vi "FaceLandmarkToPoints.vi"(8 "error in (no error)":errorcluster, 11 "FaceLandmark":refnum<k24>) -> (0 "error out":errorcluster, 2 "FaceLandmarkArray":cluster{"item":T1, T2[]}[][](array[cluster]) {"item" items=["Chin", "LeftEyebrow", "RightEyebrow", "NoseBridge", "NoseTip", "LeftEye", "RightEye", "TopLip", "BottomLip", "Nose"]; "?"."Y" format="%.2f"; "?"."X" format="%.2f"})   [LabVIEW 2020, in "FaceRecognitionDotNet.lvlib" / "FaceRecognition.lvclass"]
uses:
  FaceRecognition.lvclass
  ctl/FacePart.ctl
  ctl/Point.ctl
  dll/FaceRecognitionDotNet.dll
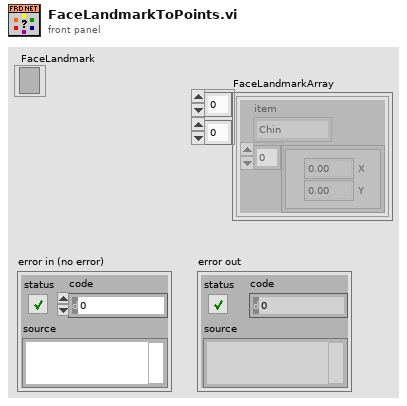
[diagram p1: front panel]
types:
  T1 = typedef "FaceRecognitionDotNet.lvlib/FaceRecognition.lvclass/FacePart.ctl" = i32
  T2 = typedef "FaceRecognitionDotNet.lvlib/FaceRecognition.lvclass/Point.ctl" = cluster{"X":sgl, "Y":sgl}
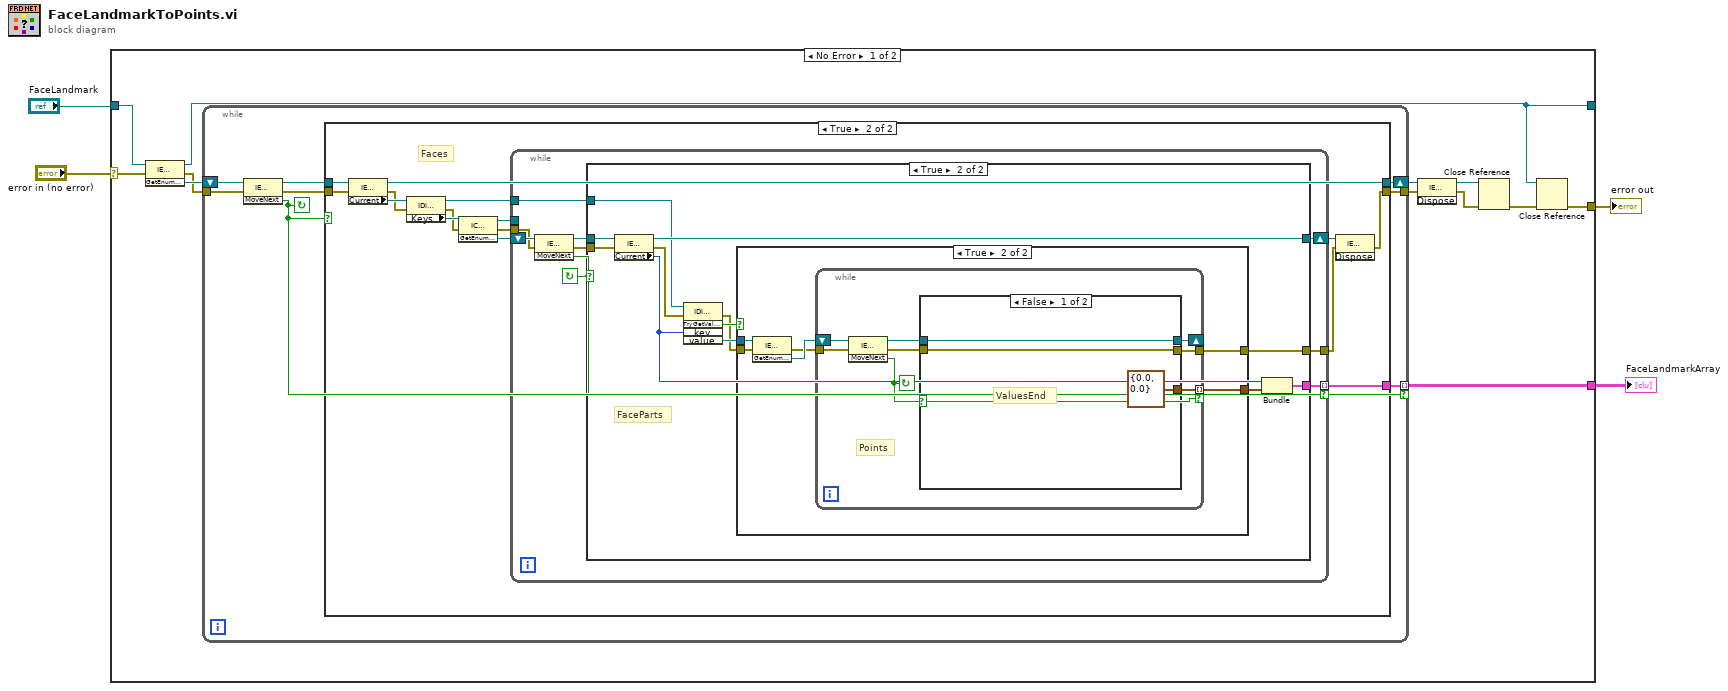
[diagram p0: block diagram]
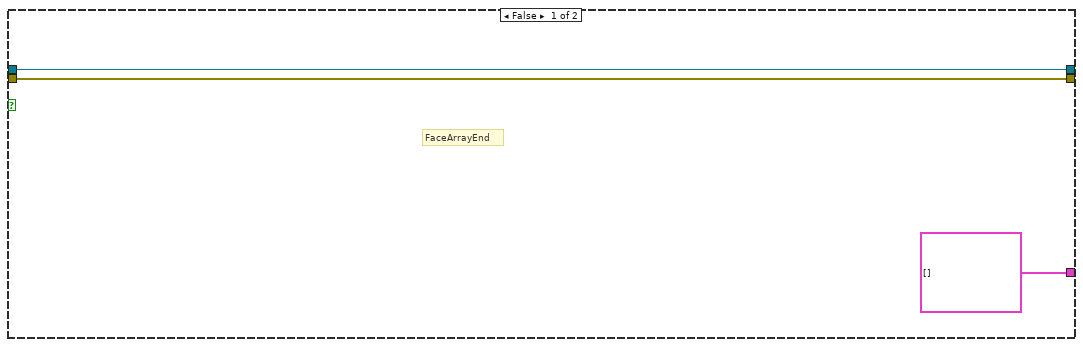
[diagram p2: hidden frame]
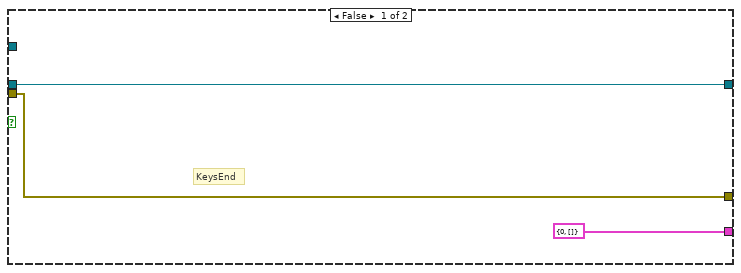
[diagram p3: hidden frame]
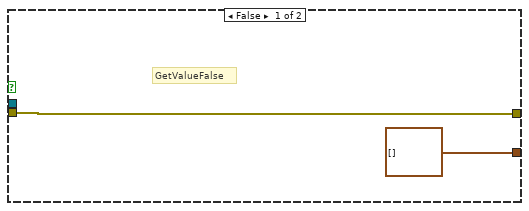
[diagram p4: hidden frame]
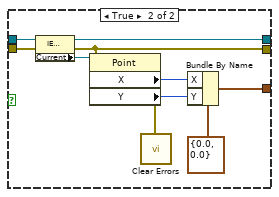
[diagram p5: hidden frame]
diagram:
  n1 = case shown="No Error" "error in (no error)" {
    selector: "error in (no error)" -> [w6 w97]
    tunnel: "FaceLandmark" -> [w16 w96]
    tunnel: [w13 _] -> w3
    tunnel: [w7 w97] -> w2
    tunnel: [w5 w96] -> _
    frame No Error {
      n2 = invoke class="IEnumerable`1[[System.Collectio" method="GetEnumerator"(reference=w16, error in=w6) -> (reference out=w5:refnum<k24>, error out=w14:errorcluster, "GetEnumerator"=w15:refnum<k24>)  [unwired: 1 in]
      n3 = while {
        tunnel: w14 -> [w21]
        shift-right: [w20] -> w12
        shift-left: w15 -> [w24]
        tunnel: [w19] -> w13 mode=indexing if=w18
        tunnel: [w17] -> w11
        stop <- w18 continue-if-true
        n4 = invoke class="IEnumerator`1[[System.Collectio" method="MoveNext"(reference=w24, error in=w21) -> (reference out=w23:refnum<k24>, error out=w22:errorcluster, "MoveNext"=w18:bool)  [unwired: 1 in]
        n5 = case shown="True" w18 {
          tunnel: w23 -> [w27 w42]
          tunnel: w22 -> [w25 w41]
          tunnel: [w27 w32] -> w20
          tunnel: [cluster{"item":i32, T2[]}[] [] w34] -> w19
          tunnel: [w25 w28] -> w17
          frame False {
            # "FaceArrayEnd"
          }
          frame True {
            # "Faces"
            n6 = property class="IEnumerator`1[[System.Collectio"(reference=w42, error in=w41) -> (reference out=w32:refnum<k24>, error out=w39:errorcluster, "Current"=w40:refnum<k24>)
            n7 = property class="IDictionary`2[[FaceRecognitionD"(reference=w40, error in=w39) -> (reference out=w33:refnum<k24>, error out=w35:errorcluster, "Keys"=w38:refnum<k24>)
            n8 = invoke class="ICollection`1[[FaceRecognitionD" method="GetEnumerator"(reference=w38, error in=w35) -> (reference out=w31:refnum<k24>, error out=w36:errorcluster, "GetEnumerator"=w37:refnum<k24>)  [unwired: 1 in]
            n9 = while {
              tunnel: w36 -> [w49]
              shift-right: [w47] -> w30
              shift-left: w37 -> [w51]
              tunnel: [w45] -> w34 mode=indexing if=w46
              tunnel: [w44] -> w29
              tunnel: w33 -> [w43]
              tunnel: w31 -> [_]
              stop <- w46 continue-if-true
              n10 = invoke class="IEnumerator`1[[FaceRecognitionD" method="MoveNext"(reference=w51, error in=w49) -> (reference out=w50:refnum<k24>, error out=w48:errorcluster, "MoveNext"=w46:bool)  [unwired: 1 in]
              n11 = case shown="True" w46 {
                tunnel: w50 -> [w54 w66]
                tunnel: w48 -> [w52 w65]
                tunnel: [w54 w64] -> w47
                tunnel: w43 -> [_ w63]
                tunnel: [cluster{"Current":i32, T2[]} {"Current"=0, []} w56] -> w45
                tunnel: [w52 w55] -> w44
                frame False {
                  # "KeysEnd"
                }
                frame True {
                  # "FaceParts"
                  n12 = property class="IEnumerator`1[[FaceRecognitionD"(reference=w66, error in=w65) -> (reference out=w64:refnum<k24>, error out=w62:errorcluster, "Current"=w57:i32)
                  n13 = invoke class="IDictionary`2[[FaceRecognitionD" method="TryGetValue"(reference=w63, error in=w62, "key"=w57) -> (error out=w59:errorcluster, "TryGetValue"=w60:bool, "value"=w61:refnum<k24>)  [unwired: 2 in, 2 out]
                  n14 = case shown="True" w60 {
                    tunnel: w61 -> [_ w74]
                    tunnel: [T2[] [] w69] -> w58
                    tunnel: w59 -> [w67 w71]
                    tunnel: [w67 w70] -> w55
                    frame False {
                      # "GetValueFalse"
                    }
                    frame True {
                      n15 = invoke class="IEnumerable`1[[FaceRecognitionD" method="GetEnumerator"(reference=w74, error in=w71) -> (error out=w72:errorcluster, "GetEnumerator"=w73:refnum<k24>)  [unwired: 1 in, 1 out]
                      n16 = while {
                        shift-right: [w80] -> _
                        shift-left: w73 -> [w82]
                        tunnel: w72 -> [w79]
                        tunnel: [w77] -> w70
                        tunnel: [w76] -> w69 mode=indexing if=w75
                        stop <- w75 continue-if-true
                        # "Points"
                        n17 = invoke class="IEnumerator`1[[FaceRecognitionD" method="MoveNext"(reference=w82, error in=w79) -> (reference out=w81:refnum<k24>, error out=w78:errorcluster, "MoveNext"=w75:bool)  [unwired: 1 in]
                        n18 = case shown="False" w75 {
                          tunnel: w81 -> [w84 w95]
                          tunnel: [w84 w90] -> w80
                          tunnel: w78 -> [w85 w89]
                          tunnel: [w85 w88] -> w77
                          tunnel: [T2 {"X"=0.0, "Y"=0.0} ("Point") w87] -> w76
                          frame False {
                            # "ValuesEnd"
                          }
                          frame True {
                            n19 = property class="IEnumerator`1[[FaceRecognitionD"(reference=w95, error in=w89) -> (reference out=w90:refnum<k24>, error out=w88:errorcluster, "Current"=w94:refnum<k24>)
                            n20 = property class="Point"(reference=w94, error in=w88) -> (error out=w86:errorcluster, "X"=w93:i32, "Y"=w92:i32)  [unwired: 1 out]
                            n21 = call <vilib>:"Clear Errors.vi"("error in (no error)"=w86) -> ()  [unwired: 5 in, 2 out]
                            n22 = Bundle By Name(cluster=T2 {"X"=0.0, "Y"=0.0} ("Point"), "X"=w93, "Y"=w92) -> (w87:T2)
                          }
                        }
                      }
                    }
                  }
                  n23 = Bundle("Current"=w57, w58) -> (w56:cluster{"Current":i32, T2[]})  [unwired: 1 in]
                }
              }
            }
            n24 = invoke class="IEnumerator`1[[FaceRecognitionD" method="Dispose"(reference=w30, error in=w29) -> (error out=w28:errorcluster)  [unwired: 1 in, 2 out]
          }
        }
      }
      n25 = invoke class="IEnumerator`1[[System.Collectio" method="Dispose"(reference=w12, error in=w11) -> (reference out=w10:refnum<k24>, error out=w9:errorcluster)  [unwired: 1 in, 1 out]
      n26 = Close Reference(reference=w10, error in (no error)=w9) -> (error out=w8:errorcluster)
      n27 = Close Reference(reference=w5, error in (no error)=w8) -> (error out=w7:errorcluster)
    }
    frame Error {
    }
  }
  "error out" <- w2
  "FaceLandmarkArray" <- w3
